vi "vai_volta_re.vi"() -> ()   [LabVIEW 2016]
uses:
  <vilib>/NXT/Subs/LVHSConnector.ctl
  <vilib>/NXT/LegoClasses/BrickReference/BrickReference.lvclass
  <vilib>/NXT/Block Support/NXT_OutputPort.ctl
  <vilib>/NXT/Block Support/NXT_InputPort.ctl
  <vilib>/NXT/Dual Mode Library/Motors/ResetMotor.vi
  <vilib>/NXT/Dual Mode Library/Motors/Rotation.vi
  <vilib>/NXT/Dual Mode Library/Sensors/Touch_Pressed.vi
  <vilib>/NXT/Dual Mode Library/Display/drawNumber.vi
  <vilib>/NXT/NXTIO Xnodes/AddressXNode/NXTIOAddress.xnode
panel:
  in  "KE 2":dbl=-0.0356
  out "NXT/EV3 3":T1
  in  "KE":dbl=-0.0356
  in  "NXT/EV3":T1
  out "Angle of Rotation":i32
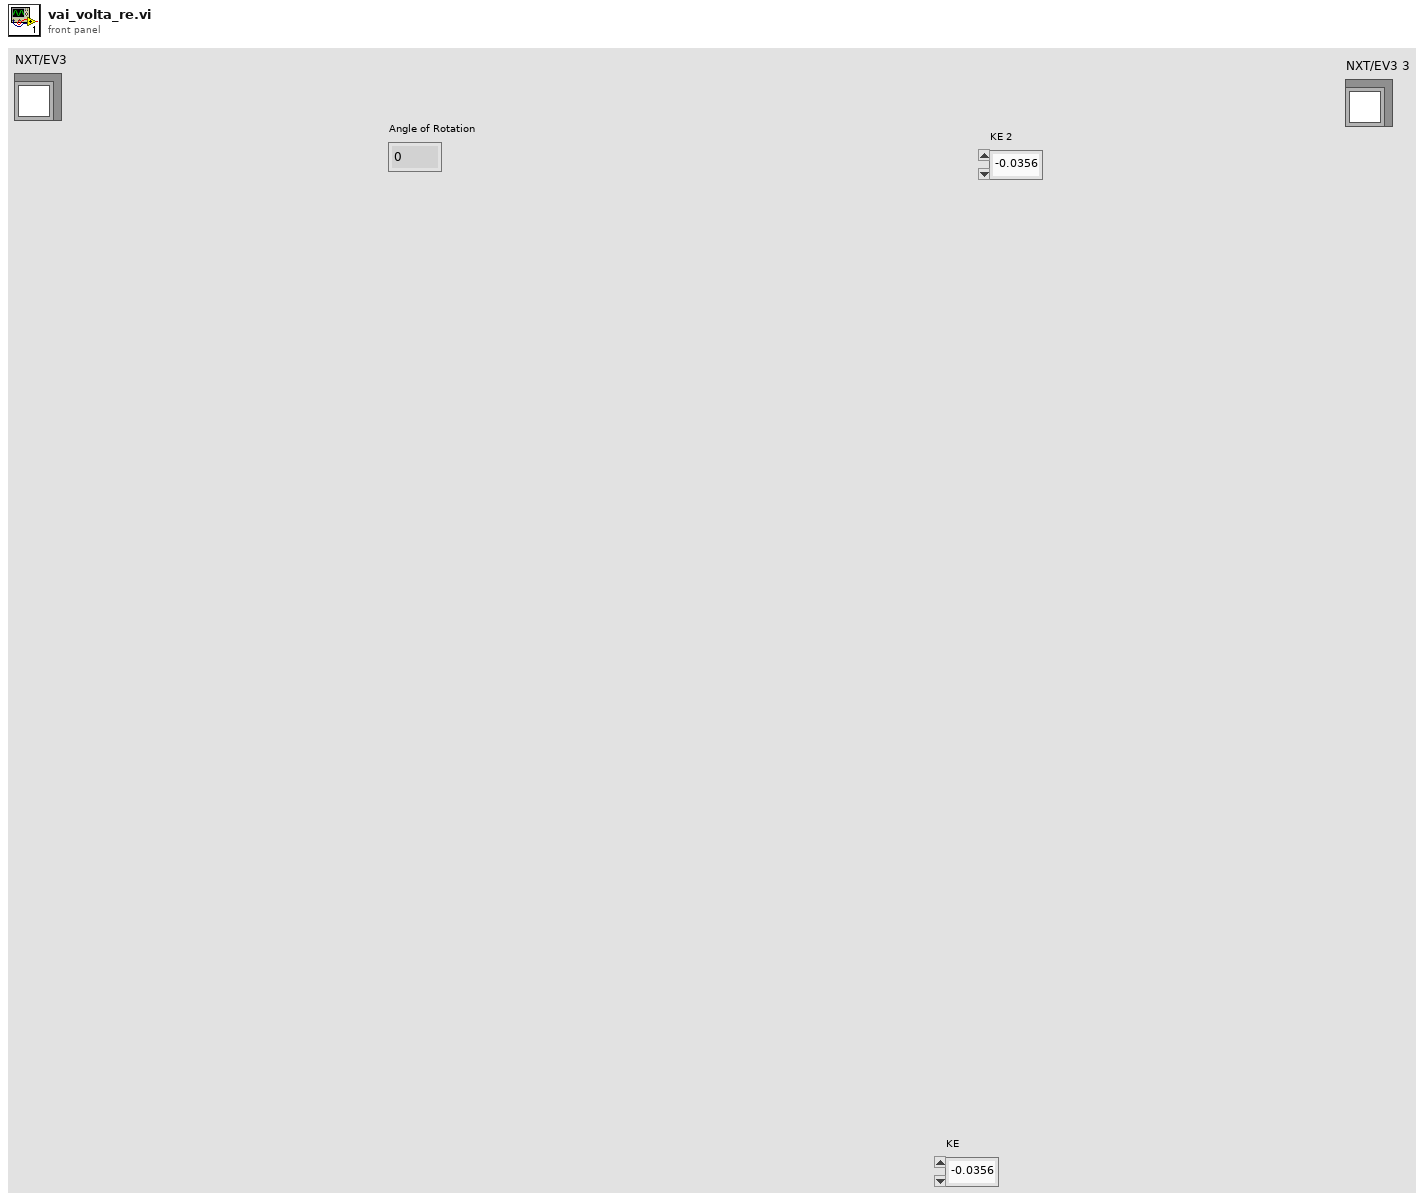
[diagram p1: front panel]
types:
  T1 = typedef "LVHSConnector.ctl" = refnum<class "BrickReference.lvclass">
  T2 = typedef "NXT_OutputPort.ctl" = u8
  T3 = typedef "NXT_InputPort.ctl" = u32
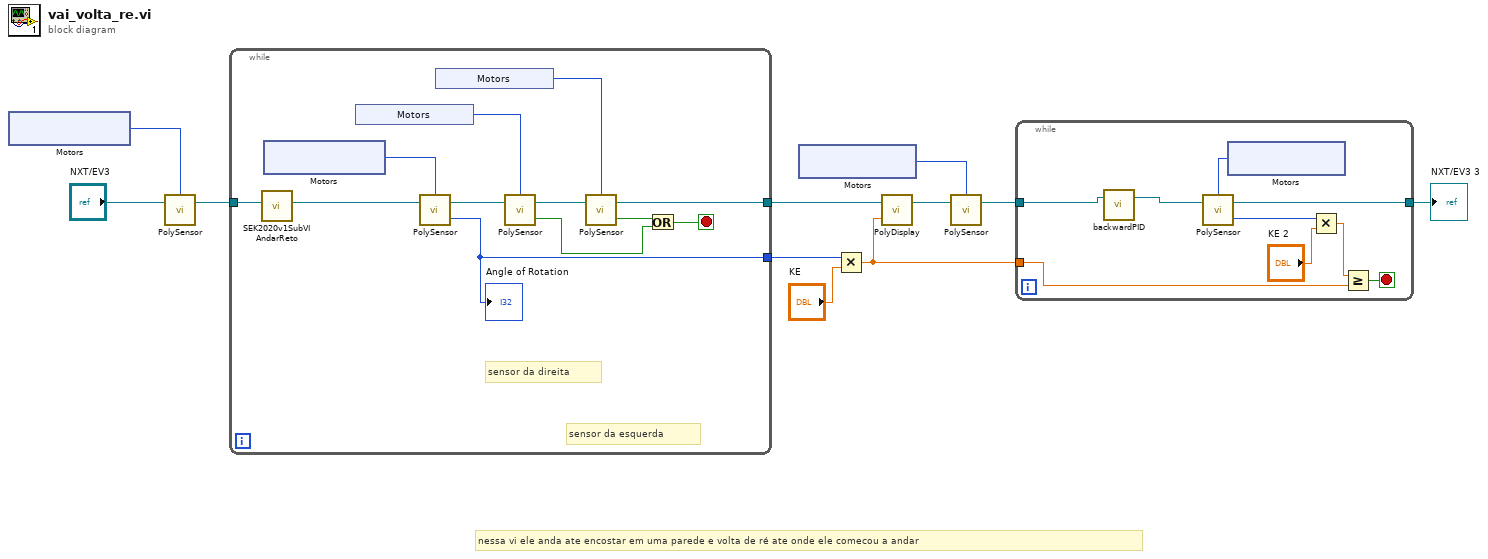
[diagram p0: block diagram]
diagram:
  # "nessa vi ele anda ate encostar em uma parede e volta de ré ate onde ele comecou a andar"
  n1 = xnode "Motors"() -> ("Motor"=w9:T2)
  n2 = call-poly <vilib>:"PolySensor.vi"("NXT/EV3"="NXT/EV3", "Port (All Ports)"=w9) -> ("NXT/EV3"=w8:T1)  [unwired: 2 out]
  n3 = while {
    tunnel: w8 -> [w14]
    tunnel: [w15] -> w10
    tunnel: [w23] -> w6
    stop <- w17 stop-if-true
    # "sensor da esquerda"
    # "sensor da direita"
    n4 = call "SEK2020v1SubVIAndarReto.vi"("NXT/EV3"=w14) -> ("NXT/EV3 2"=w13:T1)  [unwired: 9 in]
    n5 = xnode "Motors"() -> ("Motor"=w12:T2)
    n6 = xnode "Motors"() -> ("Sensor"=w21:T3)
    n7 = call-poly <vilib>:"PolySensor.vi"("NXT/EV3"=w13, "Port (Port A)"=w12) -> ("Angle of Rotation"=w23:i32, "NXT/EV3"=w16:T1)  [unwired: 1 out]
    "Angle of Rotation" <- w23
    n8 = xnode "Motors"() -> ("Sensor"=w20:T3)
    n9 = call-poly <vilib>:"PolySensor.vi"("NXT/EV3"=w16, "Port (Port 1)"=w21) -> ("Yes / No"=w18:bool, "NXT/EV3"=w22:T1)  [unwired: 1 in]
    n10 = call-poly <vilib>:"PolySensor.vi"("NXT/EV3"=w22, "Port (Port 1)"=w20) -> ("Yes / No"=w19:bool, "NXT/EV3"=w15:T1)  [unwired: 1 in]
    n11 = Or(x=w19, y=w18) -> (x .or. y?=w17:bool)
  }
  n12 = xnode "Motors"() -> ("Motor"=w5:T2)
  n13 = Multiply(x=w6, y="KE") -> (x*y=w1:dbl)
  n14 = call-poly <vilib>:"PolyDisplay.vi"("number"=w1, "NXT/EV3"=w10) -> ("NXT/EV3"=w2:T1)  [unwired: 2 in]
  n15 = call-poly <vilib>:"PolySensor.vi"("NXT/EV3"=w2, "Port (All Ports)"=w5) -> ("NXT/EV3"=w4:T1)  [unwired: 2 out]
  n16 = while {
    tunnel: w4 -> [w28]
    tunnel: [w35] -> w3
    tunnel: w1 -> [w29]
    stop <- w34 stop-if-true
    n17 = call "backwardPID.vi"("NXT/EV3"=w28) -> ("NXT/EV3 2"=w27:T1)  [unwired: 2 in]
    n18 = xnode "Motors"() -> ("Motor"=w33:T2)
    n19 = call-poly <vilib>:"PolySensor.vi"("NXT/EV3"=w27, "Port (Port A)"=w33) -> ("Angle of Rotation"=w32:i32, "NXT/EV3"=w35:T1)  [unwired: 1 out]
    n20 = Multiply(x=w32, y="KE 2") -> (x*y=w31:dbl)
    n21 = Greater Or Equal?(x=w31, y=w29) -> (x >= y?=w34:bool)
  }
  "NXT/EV3 3" <- w3
